vi "main.vi"() -> ()   [LabVIEW 2025]
uses:
  <vilib>/DAQmx/write.llb/DAQmx Write (Analog 1D DBL 1Chan NSamp).vi
  <vilib>/Analysis/2dsp.llb/Power Spectrum (DBL).vi
  <vilib>/DAQmx/read.llb/DAQmx Read (Analog 1D DBL 1Chan NSamp).vi
  <vilib>/DAQmx/create/channels.llb/DAQmx Create Channel (AO-Voltage-Basic).vi
  <vilib>/DAQmx/configure/timing.llb/DAQmx Timing (Sample Clock).vi
  <vilib>/DAQmx/create/channels.llb/DAQmx Create Channel (AI-Voltage-Basic).vi
  <vilib>/DAQmx/miscellaneous.llb/DAQmx Fill In Error Info.vi
  <vilib>/Analysis/NI_AAL_SigProc.lvlib
  <vilib>/Analysis/NI_AALPro.lvlib
panel:
  out "Detected Frequency (Hz)":dbl
  in  "stop":bool
  out "Frequency OK":bool
  out "FFT Spectrum":waveform(dbl)(graph)
  out "Acquired Signal":dbl[](graph)
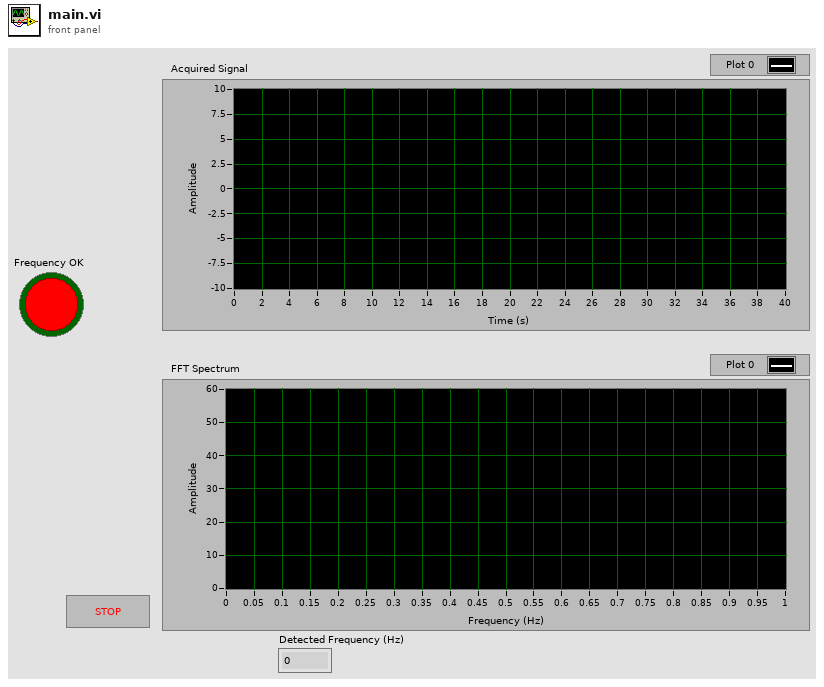
[diagram p1: front panel]
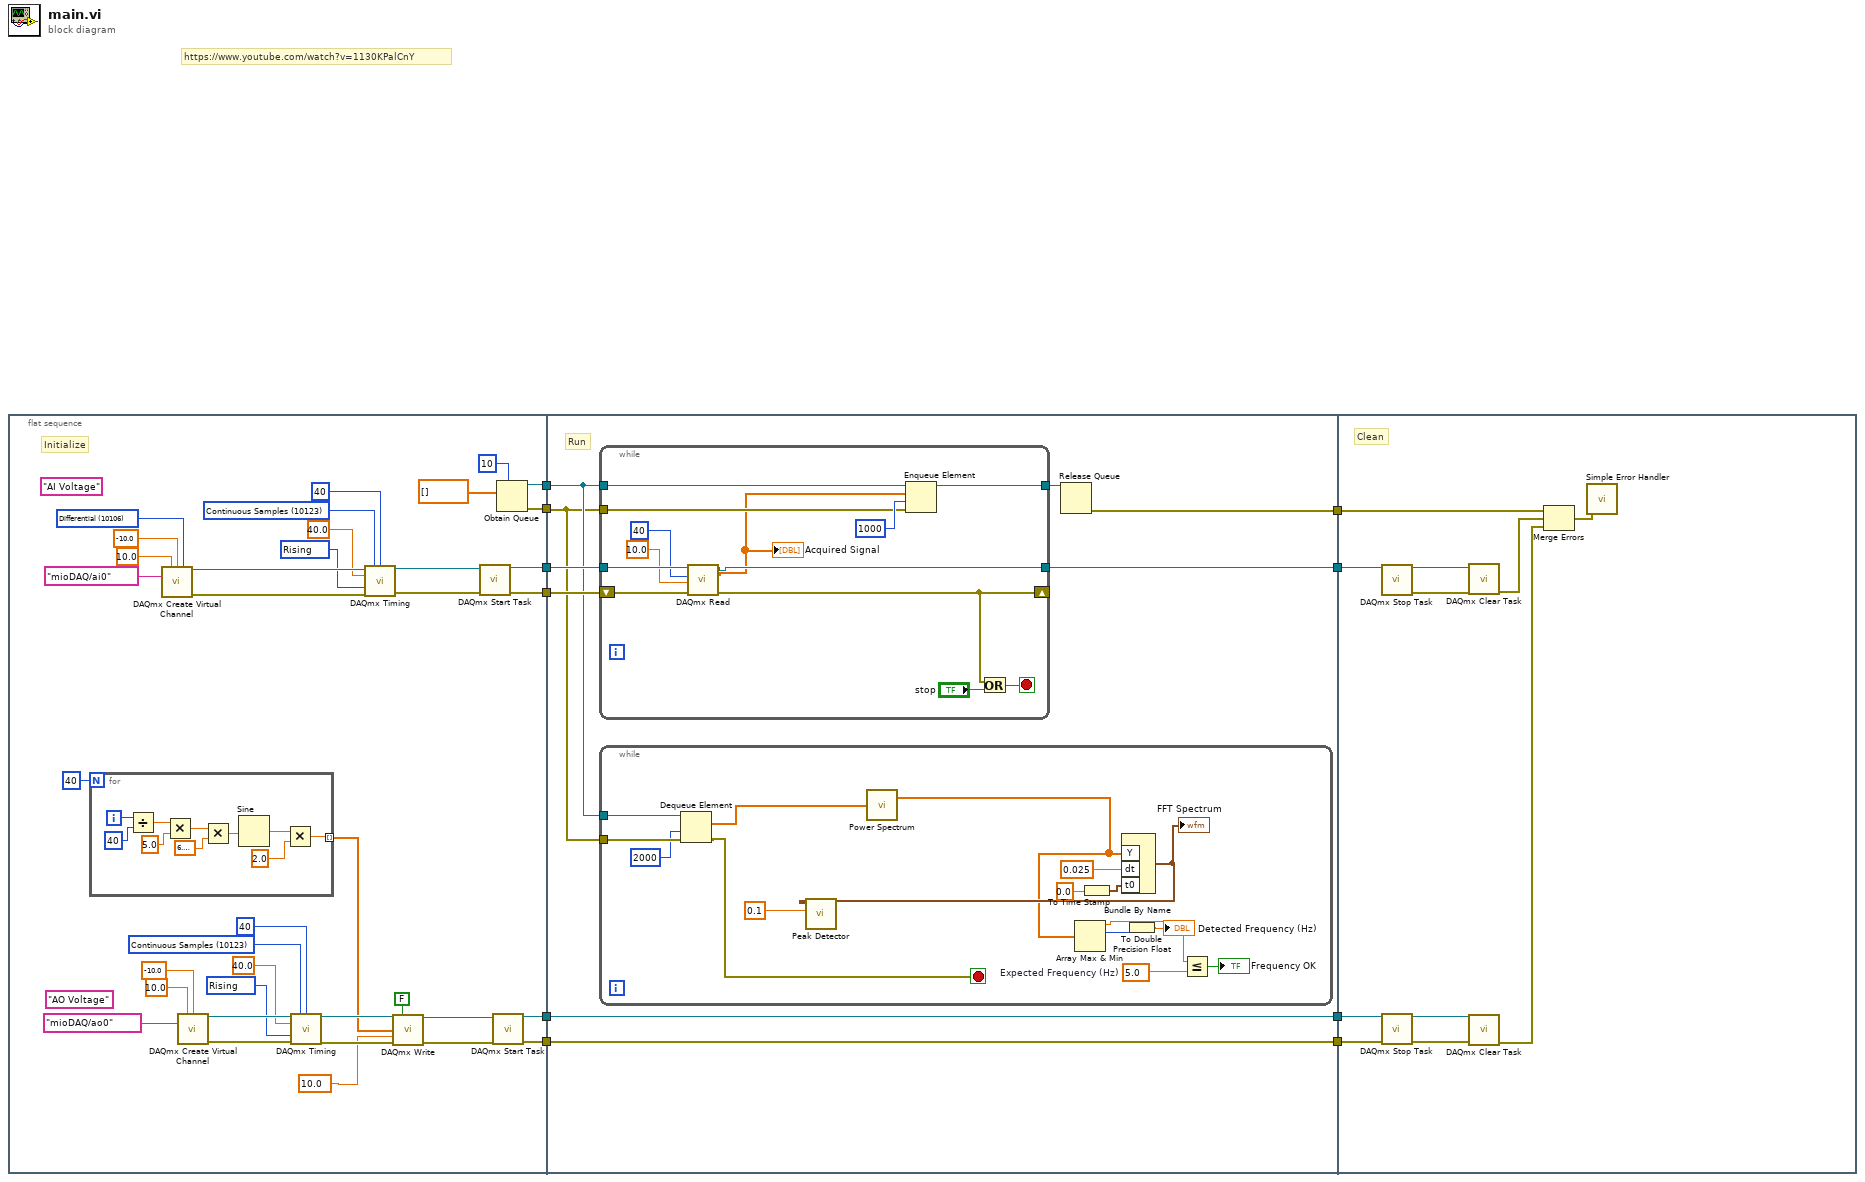
[diagram p0: block diagram]
diagram:
  # "https://www.youtube.com/watch?v=1130KPalCnY"
  n1 = flat-sequence {
    tunnel: [w47] -> w10
    tunnel: [w18] -> w9
    tunnel: [w17] -> w8
    tunnel: [w14] -> w7
    tunnel: [w13] -> w4
    tunnel: [w12] -> w3
    tunnel: w10 -> [w63]
    tunnel: w9 -> [w65]
    tunnel: w8 -> [w64]
    tunnel: w7 -> [w62]
    tunnel: [w61] -> w6
    tunnel: [w60] -> w5
    tunnel: w4 -> [w60]
    tunnel: w3 -> [w59]
    tunnel: [w59] -> w2
    tunnel: [w58] -> w1
    tunnel: w6 -> [w99]
    tunnel: w5 -> [w98]
    tunnel: w2 -> [w97]
    tunnel: w1 -> [w96]
    frame #0 {
      (unwired) "AI Voltage" ("new task name")
      w26 = 10123 items=["Finite Samples"=10178, "Continuous Samples"=10123, "Hardware Timed Single Point"=12522] ("sample mode")
      w23 = 10280 items=["Rising"=10280, "Falling"=10171] ("active edge")
      w20 = 10106 items=["Default"=-1, "RSE"=10083, "NRSE"=10078, "Differential"=10106, "Pseudodifferential"=12529] ("input terminal configuration")
      w39 = 10123 items=["Finite Samples"=10178, "Continuous Samples"=10123, "Hardware Timed Single Point"=12522] ("sample mode")
      w40 = 10280 items=["Rising"=10280, "Falling"=10171] ("active edge")
      (unwired) "AO Voltage" ("new task name")
      # "Initialize"
      n2 = for {
        N: 40 -> [_]
        tunnel: [w48] -> w34 mode=indexing
        i -> [w56]
        n3 = Divide(x=w56, y=40) -> (x/y=w55:dbl)
        n4 = Multiply(x=w55, y=5.0) -> (x*y=w53:dbl)
        n5 = Multiply(x=w53, y=6.283185307179586) -> (x*y=w51:dbl)
        n6 = Sine(x=w51) -> (sin(x)=w50:dbl)
        n7 = Multiply(x=w50, y=2.0) -> (x*y=w48:dbl)
      }
      n8 = call-poly <vilib>:"DAQmx Create Virtual Channel.vi"("maximum value"=10.0, "minimum value"=-10.0, "input terminal configuration"=w20, "physical channels"=tag "mioDAQ/ai0") -> ("task out"=w27:refnum<k21>, "error out"=w28:errorcluster)  [unwired: 10 in]
      n9 = call-poly <vilib>:"DAQmx Create Virtual Channel.vi"("maximum value"=10.0, "minimum value"=-10.0, "physical channels"=tag "mioDAQ/ao0") -> ("task out"=w42:refnum<k21>, "error out"=w43:errorcluster)  [unwired: 11 in]
      n10 = call-poly <vilib>:"DAQmx Timing.vi"("task/channels in"=w42, "sample mode"=w39, "samples per channel"=40, "rate"=40.0, "active edge"=w40, "error in"=w43) -> ("task out"=w36:refnum<k21>, "error out"=w35:errorcluster)  [unwired: 8 in]
      n11 = call-poly <vilib>:"DAQmx Timing.vi"("task/channels in"=w27, "sample mode"=w26, "samples per channel"=40, "rate"=40.0, "active edge"=w23, "error in"=w28) -> ("task out"=w29:refnum<k21>, "error out"=w30:errorcluster)  [unwired: 8 in]
      n12 = call-poly <vilib>:"DAQmx Write.vi"("task/channels in"=w36, "auto start"=FALSE, "data"=w34, "timeout"=10.0, "error in"=w35) -> ("task out"=w32:refnum<k21>, "error out"=w31:errorcluster)  [unwired: 8 in, 1 out]
      n13 = call <vilib>:"DAQmx Start Task.vi"("task/channels in"=w29, "error in"=w30) -> ("task out"=w18:refnum<k21>, "error out"=w17:errorcluster)  [unwired: 12 in]
      n14 = call <vilib>:"DAQmx Start Task.vi"("task/channels in"=w32, "error in"=w31) -> ("task out"=w13:refnum<k21>, "error out"=w12:errorcluster)  [unwired: 12 in]
      n15 = Obtain Queue(max queue size (-1, unlimited)=10, element data type=dbl[] [] ("timeout")) -> (queue out=w47:refnum<queue>, error out=w14:errorcluster)  [unwired: 3 in, 1 out]
    }
    frame #1 {
      # "Run"
      n16 = while {
        tunnel: [w95] -> w66
        tunnel: w63 -> [w94]
        tunnel: w65 -> [w92]
        shift-right: [w87] -> _
        shift-left: w64 -> [w91]
        tunnel: w62 -> [w85]
        tunnel: [w84] -> w61
        stop <- w93 stop-if-true
        n17 = call-poly <vilib>:"DAQmx Read.vi"("task/channels in"=w92, "number of samples per channel"=40, "timeout"=10.0, "error in"=w91) -> ("task out"=w84:refnum<k21>, "data"=w83:dbl[], "error out"=w87:errorcluster)  [unwired: 9 in]
        "Acquired Signal" <- w83
        n18 = Enqueue Element(queue=w94, element=w83, timeout in ms (-1)=1000, error in (no error)=w85) -> (queue out=w95:refnum<queue>)  [unwired: 2 out]
        n19 = Or(x=w87, y="stop") -> (x .or. y?=w93:bool)
      }
      n20 = while {
        tunnel: w63 -> [w82]
        tunnel: w62 -> [w81]
        stop <- w76 stop-if-true
        w72 = 5.0  # Expected Frequency (Hz)
        n21 = Dequeue Element(queue=w82, timeout in ms (-1)=2000, error in (no error)=w81) -> (element=w68:dbl[], error out=w76:errorcluster)  [unwired: 2 out]
        n22 = call-poly <vilib>:"Power Spectrum.vi"("X"=w68) -> ("Power Spectrum"=w67:dbl[])  [unwired: 1 out]
        n23 = Array Max & Min(array=w67) -> (max value=w70:dbl, max index (indices)=w74:i32)  [unwired: 2 out]
        n24 = To Time Stamp(1:0.0 ("dt")) -> (0:w77:timestamp)
        n25 = Bundle By Name("Y"=w67, "dt"=0.025, "t0"=w77) -> (w69:waveform(dbl))  [unwired: 1 in]
        "FFT Spectrum" <- w69
        n26 = call <vilib>:"Peak Detector.vi"("threshold"=0.1, "X"=w69) -> ()  [unwired: 5 in, 5 out]
        n27 = To Double Precision Float(number=w74) -> (double precision float=→"Detected Frequency (Hz)":dbl)
        n28 = Less Or Equal?(x=w70, y=w72) -> (x <= y?=→"Frequency OK":bool)
      }
      n29 = Release Queue(queue=w66) -> (error out=w58:errorcluster)  [unwired: 2 in, 2 out]
    }
    frame #2 {
      # "Clean"
      n30 = call <vilib>:"DAQmx Stop Task.vi"("task/channels in"=w99) -> ("task out"=w106:refnum<k21>, "error out"=w105:errorcluster)  [unwired: 13 in]
      n31 = call <vilib>:"DAQmx Stop Task.vi"("task/channels in"=w98, "error in"=w97) -> ("task out"=w104:refnum<k21>, "error out"=w103:errorcluster)  [unwired: 12 in]
      n32 = call <vilib>:"DAQmx Clear Task.vi"("task in"=w106, "error in"=w105) -> ("error out"=w101:errorcluster)  [unwired: 13 in]
      n33 = call <vilib>:"DAQmx Clear Task.vi"("task in"=w104, "error in"=w103) -> ("error out"=w100:errorcluster)  [unwired: 13 in]
      n34 = Merge Errors(w96, w101, w100) -> (w102:errorcluster)
      n35 = call <vilib>:"Simple Error Handler.vi"("error in (no error)"=w102) -> ()  [unwired: 4 in, 5 out]
    }
  }
